vi "RFH-convert-r140andLibreVNA.vi"() -> ()   [LabVIEW 2020, in "RFH-Reflection_File_Handler.lvlib"]
uses:
  RFH-Reflection_File_Handler.lvlib
panel:
  out "error out LibreVNA":errorcluster
  out "error out R140":errorcluster
  in  "destionation path":path
  in  "All libreVNA data folder":path
  in  "R140 Excel files":path
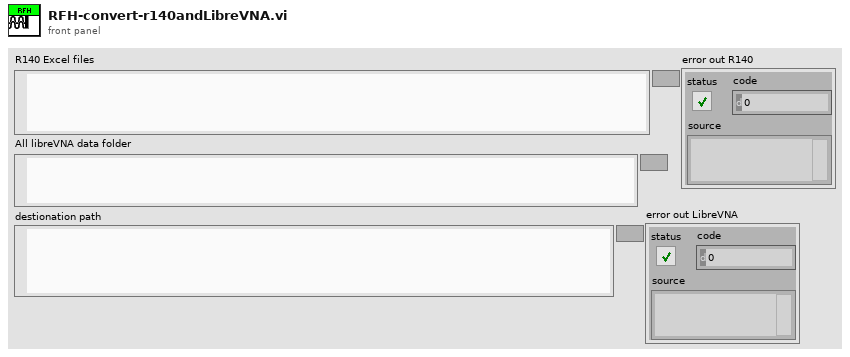
[diagram p1: front panel]
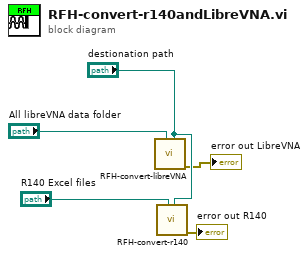
[diagram p0: block diagram]
diagram:
  n1 = call "RFH-convert-libreVNA.vi"("destionation path"="destionation path", "All libreVNA data folder"="All libreVNA data folder") -> ("error out"=→"error out LibreVNA":errorcluster)  [unwired: 9 in]
  n2 = call "RFH-convert-r140.vi"("Destination Folder"="destionation path", "Folder Path"="R140 Excel files") -> ("error out"=→"error out R140":errorcluster)  [unwired: 9 in]
